vi "Confidence Interval using Inverse t.vi"() -> ()   [LabVIEW 2023]
doc: "Determines the next data point within a 95.45% (or any other) confidence level based on the given data. In this VI, the data represents the mean time between failures in hours."
uses:
  <vilib>/Analysis/1siggen.llb/Ramp Pattern by Samples.vi
  <vilib>/gmath/statdist.llb/Student t Inverse CDF.vi
  <vilib>/gmath/statdist.llb/Normal PDF.vi
  <vilib>/Analysis/NI_AALBase.lvlib
  <vilib>/gmath/NI_Gmath.lvlib
panel:
  out "Measurements":dbl[](array[numeric])
  out "Measurement Number":i32
  out "Scale":dbl
  out "Correction":dbl format="%#.6g"
  in  "Standard Uncertainty":dbl=0.01 format="%0.2f"
  in  "Standard Value":dbl=1000.0 format="%#.6g"
  out "Mean Value":dbl format="%#.6g"
  out "t-student coefficient":dbl
  out "Histogram Graph":cluster{"X Values":dbl[], dbl[]}[](graph)
  out "Uncertainty":dbl format="%0.2f"
  in  "Confidence Level (%)":dbl=95.45 format="%0.2f"
  out "Degrees of Freedom (n-1)":i32
  out "Mean":dbl format="%#.6g"
  out "Standard Deviation":dbl format="%0.2f"
  # "Overview: Demonstrates how to obtain the repeatability of a set of measurement samples.\nRequirements: LabVIEW Full Development System\nInstructions: \n1. Run the VI.\n2. Analyze the result of the evaluation of the uncertainty of this measurement."
  # "+"
  # "g"
  # "The Repeatability (Type A uncertainty) of this measurement is:"
  # "+"
  # "g"
  # "+"
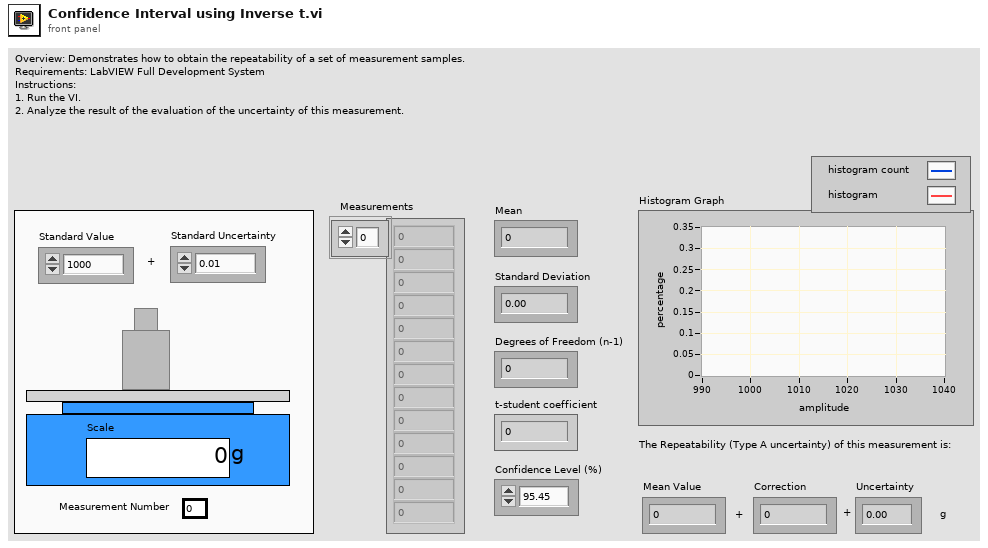
[diagram p1: front panel]
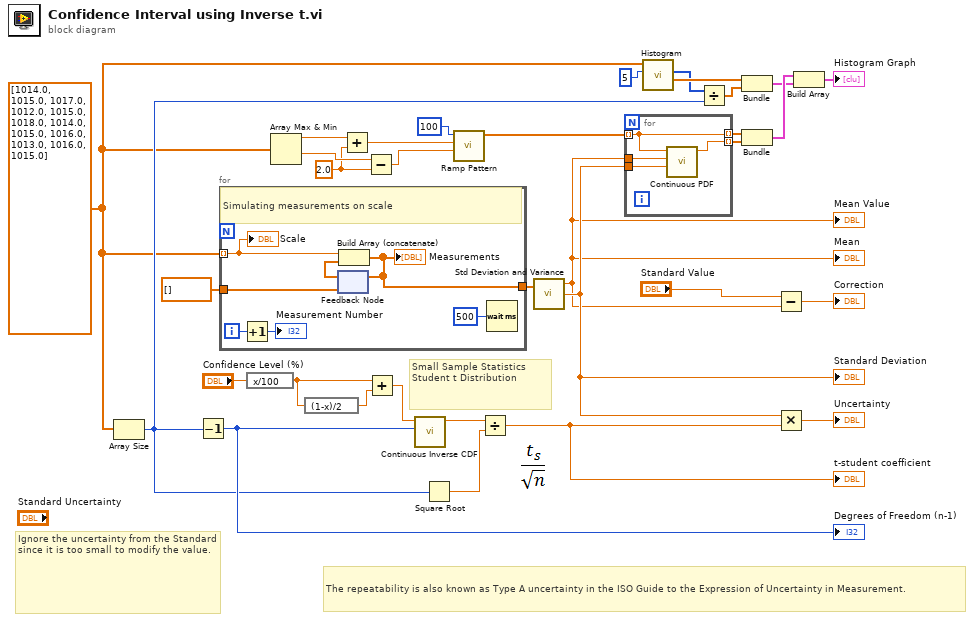
[diagram p0: block diagram]
diagram:
  w3 = dbl[] [1014.0, 1015.0, 1017.0, 1012.0, 1015.0, 1018.0, 1014.0, 1015.0, 1016.0, 1013.0, 1016.0, 1015.0] ("Samples")
  w4 = 2.0 ("y")
  # "The repeatability is also known as Type A uncertainty in the ISO Guide to the Expression of Uncertainty in Measurement."
  # "Ignore the uncertainty from the Standard since it is too small to modify the value."
  # "Small Sample Statistics\nStudent t Distribution"
  n1 = Array Size(array=w3) -> (size(s)=w10:i32)
  n2 = Decrement(x=w10) -> (x-1=w32:i32)
  "Degrees of Freedom (n-1)" <- w32
  n3 = for {
    tunnel: w3 -> [w38] mode=indexing
    tunnel: [w36] -> w2
    tunnel: dbl[] [] -> [w35]
    i -> [w40]
    # "Simulating measurements on scale"
    n4 = Increment(x=w40) -> (x+1=→"Measurement Number":i32)
    n5 = feedback #1(w35) -> (w37:dbl[])
    n6 = Build Array (concatenate)(w38, w37) -> (w36:dbl[])
    "Measurements" <- w36
    n7 = feedback-in #1(w36) -> ()
    n8 = Wait (ms)(milliseconds to wait=u32 500 ("millisecond multiple")) -> ()  [unwired: 1 out]
    "Scale" <- w38
  }
  n9 = expression code="x/100"("Confidence Level (%)") -> (w28:dbl)
  n10 = Array Max & Min(array=w3) -> (max value=w23:dbl, min value=w24:dbl)  [unwired: 2 out]
  n11 = expression code="(1-x)/2"(w28) -> (w30:dbl)
  n12 = Add(x=w23, y=w4) -> (x+y=w14:dbl)
  n13 = Subtract(x=w24, y=w4) -> (x-y=w13:dbl)
  n14 = Add(x=w28, y=w30) -> (x+y=w31:dbl)
  n15 = call-poly <vilib>:"Continuous Inverse CDF.vi"("k degrees of freedom"=w32, "cdf(x)"=w31) -> ("x"=w27:dbl)  [unwired: 8 in, 1 out]
  n16 = Square Root(x=w10) -> (sqrt(x)=w8:dbl)
  n17 = call-poly <vilib>:"Ramp Pattern.vi"("start"=w13, "end"=w14, "samples"=100) -> ("Ramp Pattern"=w21:dbl[])  [unwired: 7 in, 1 out]
  n18 = Divide(x=w27, y=w8) -> (x/y=w9:dbl)
  "t-student coefficient" <- w9
  n19 = call <vilib>:"Std Deviation and Variance.vi"("X"=w2) -> ("mean"=w5:dbl, "standard deviation"=w17:dbl)  [unwired: 1 in, 1 out]
  "Standard Deviation" <- w17
  "Mean" <- w5
  "Mean Value" <- w5
  n20 = for {
    tunnel: w5 -> [w44]
    tunnel: w17 -> [w43]
    tunnel: w21 -> [w41] mode=indexing
    tunnel: [w41] -> w20 mode=indexing
    tunnel: [w42] -> w19 mode=indexing
    n21 = call-poly <vilib>:"Continuous PDF.vi"("std"=w43, "mean"=w44, "x"=w41) -> ("pdf(x)"=w42:dbl)  [unwired: 7 in, 1 out]
  }
  n22 = call <vilib>:"Histogram.vi"("intervals"=5, "X"=w3) -> ("X Values"=w25:dbl[], "Histogram: h(x)"=w12:i32[])  [unwired: 6 in, 2 out]
  n23 = Divide(x=w12, y=w10) -> (x/y=w11:dbl[])
  n24 = Bundle("X Values"=w25, w11) -> (w15:cluster{"X Values":dbl[], dbl[]})  [unwired: 1 in]
  n25 = Bundle(w20, w19) -> (w16:cluster{dbl[], dbl[]})  [unwired: 1 in]
  n26 = Subtract(x="Standard Value", y=w5) -> (x-y=→"Correction":dbl)
  n27 = Multiply(x=w17, y=w9) -> (x*y=→"Uncertainty":dbl)
  n28 = Build Array(w16, w15) -> (→"Histogram Graph":cluster{"X Values":dbl[], dbl[]}[])
